vi "Run Frequency Response Analysis.vi"(8 "error in (no error)":errorcluster, 11 "VISA resource name":refnum<visa-resource-name>) -> (0 "error out":errorcluster, 3 "VISA resource name out":refnum<visa-resource-name>)   [LabVIEW 2023, in "Keysight-DSQx3014T.lvlib"]
doc: "Starts the frequency response analysis. When the frequency response analysis done, you can use <b>Read Frequency Response Analysis Data.vi</b> to query the data.\n\nNote: This VI is only applicable for 1000 X-Series."
uses:
  Keysight-DSQx3014T.lvlib
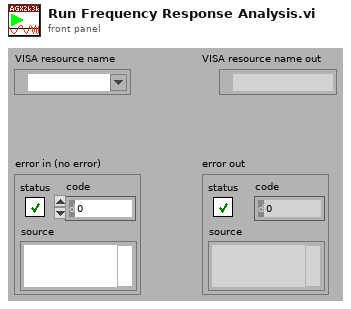
[diagram p1: front panel]
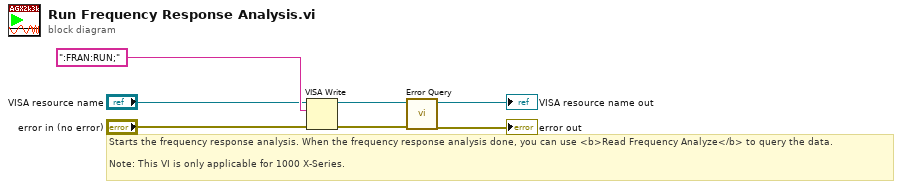
[diagram p0: block diagram]
diagram:
  # "Starts the frequency response analysis. When the frequency response analysis done, you can use <b>Read Frequency Analyze</b> to query the data.\n\nNote: This VI is only applicable for 1000 X-Series."
  n1 = VISA Write(VISA resource name="VISA resource name", write buffer=":FRAN:RUN;", error in (no error)="error in (no error)") -> (VISA resource name out=w4:refnum<visa-resource-name>, error out=w3:errorcluster)  [unwired: 1 out]
  n2 = call "Error Query.vi"("error in (no error)"=w3, "VISA resource name"=w4) -> ("error out"=→"error out":errorcluster, "VISA resource name out"=→"VISA resource name out":refnum<visa-resource-name>)  [unwired: 6 in, 2 out]
